vi "Main FPGA.vi"(7 "Motor Values":T3) -> ()   [LabVIEW 2013]
uses:
  <vilib>/rvi/Emulation/niFpgaSctlEmulationGetInTimedLoop.vi
  <vilib>/rvi/Emulation/niFpgaEmulationReportErrorSimple.vi
  <vilib>/rvi/Emulation/niFpgaGetClockAttributes.vi
  <vilib>/rvi/eio/common/nirviEmuTemplateMethod_errors.vi
  <vilib>/rvi/Emulation/niFpgaCriticalErrorInLSC.vi
  <vilib>/rvi/Emulation/niFpgaProcessEmulError.vi
  <vilib>/eio/EIONode/EIONode.xnode
panel:
  out "Data bit array":bool[](array[boolean])
  out "I2C FPGA Running":bool=TRUE
  in  "I2C Read":T1={"Data to send"=[0, 0, 0, 0, 0, 0, 0, 0], "Number of Bytes"=0, "Data to send 2"=[0, 0, 0, 0, 0, 0, 0, 0], "Number of Bytes 2"=0, "Data to send 3"=[0, 0, 0, 0, 0, 0, 0, 0], "Number of Bytes 3"=0, "Number of Bytes 4"=0, "I2C Start"=FALSE}
  in  "Position Reset 3":bool
  out "Position (Counts) 3":i16
  in  "Position Reset 2":bool
  out "Position (Counts) 2":i16
  out "Position (Counts)":i16
  in  "Position Reset":bool
  in  "Enable 4":bool
  in  "Encoder Intputs Motor 3":T2={"Tach 2"="ConnectorA/DIO9", "Tach 1"="ConnectorA/DIO8"}
  in  "Motor Values 3":T3
  in  "Motor Values 2":T3
  in  "Encoder Intputs Motor 2":T2={"Tach 2"="ConnectorB/DIO7", "Tach 1"="ConnectorB/DIO6"}
  in  "Encoder Intputs Motor 1":T2={"Tach 2"="ConnectorB/DIO9", "Tach 1"="ConnectorB/DIO8"}
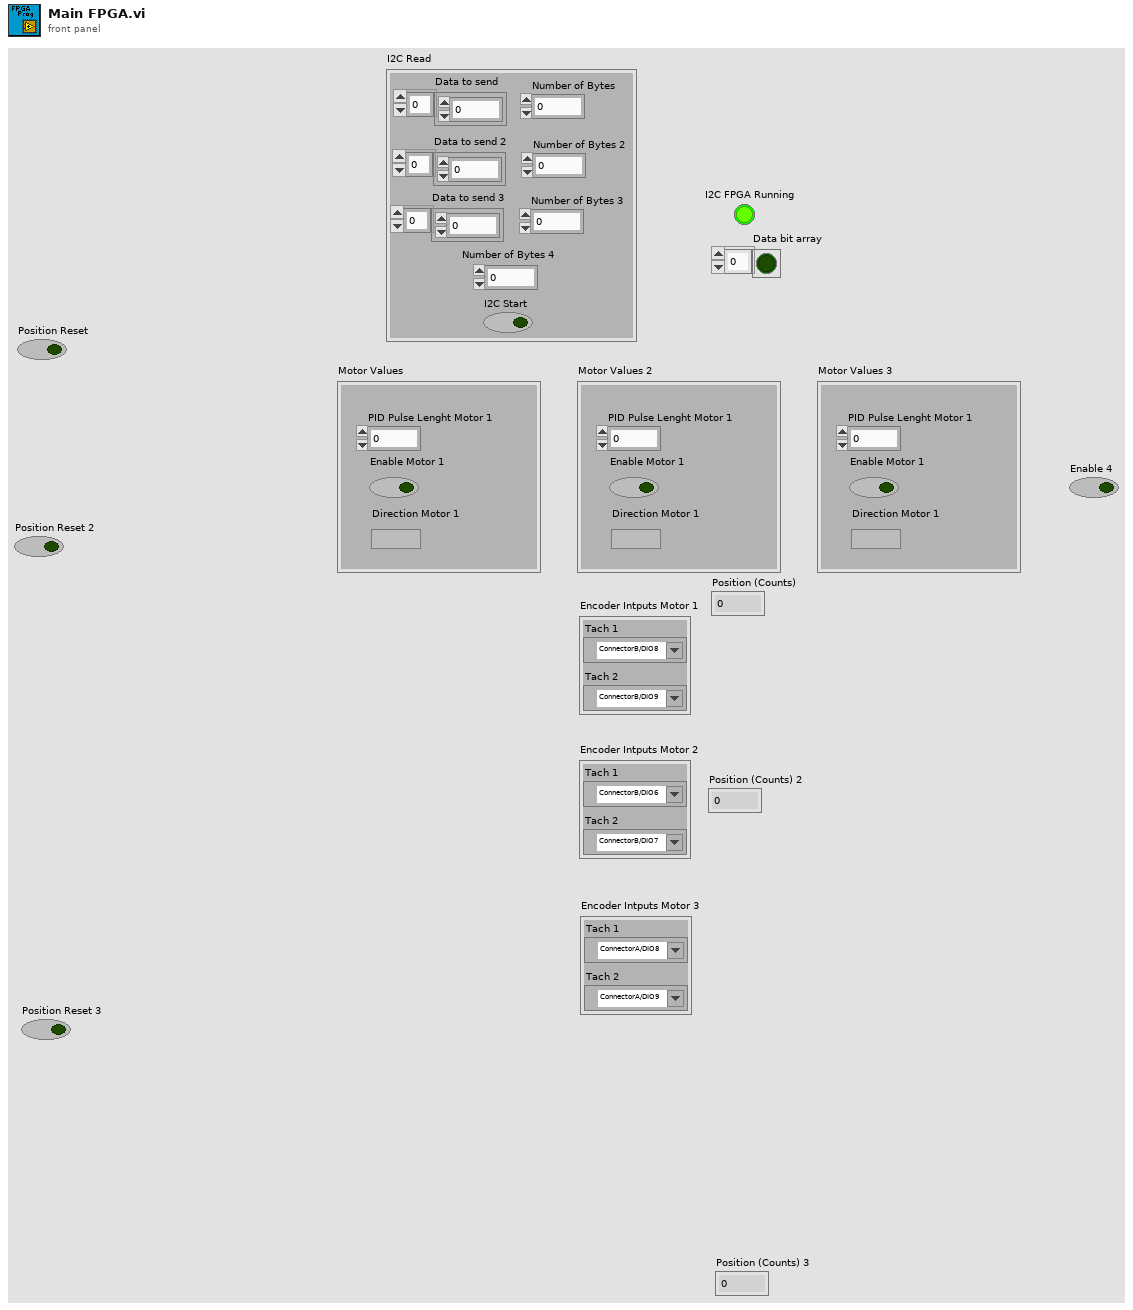
[diagram p1: front panel]
types:
  T1 = cluster{"Data to send":u8[], "Number of Bytes":i16, "Data to send 2":u8[], "Number of Bytes 2":i16, "Data to send 3":u8[], "Number of Bytes 3":i16, "Number of Bytes 4":i16, "I2C Start":bool}
  T2 = cluster{"Tach 2":refnum<k21>, "Tach 1":refnum<k21>}
  T3 = cluster{"PID Pulse Lenght Motor 1":i16, "Enable Motor 1":bool, "Direction Motor 1":bool}
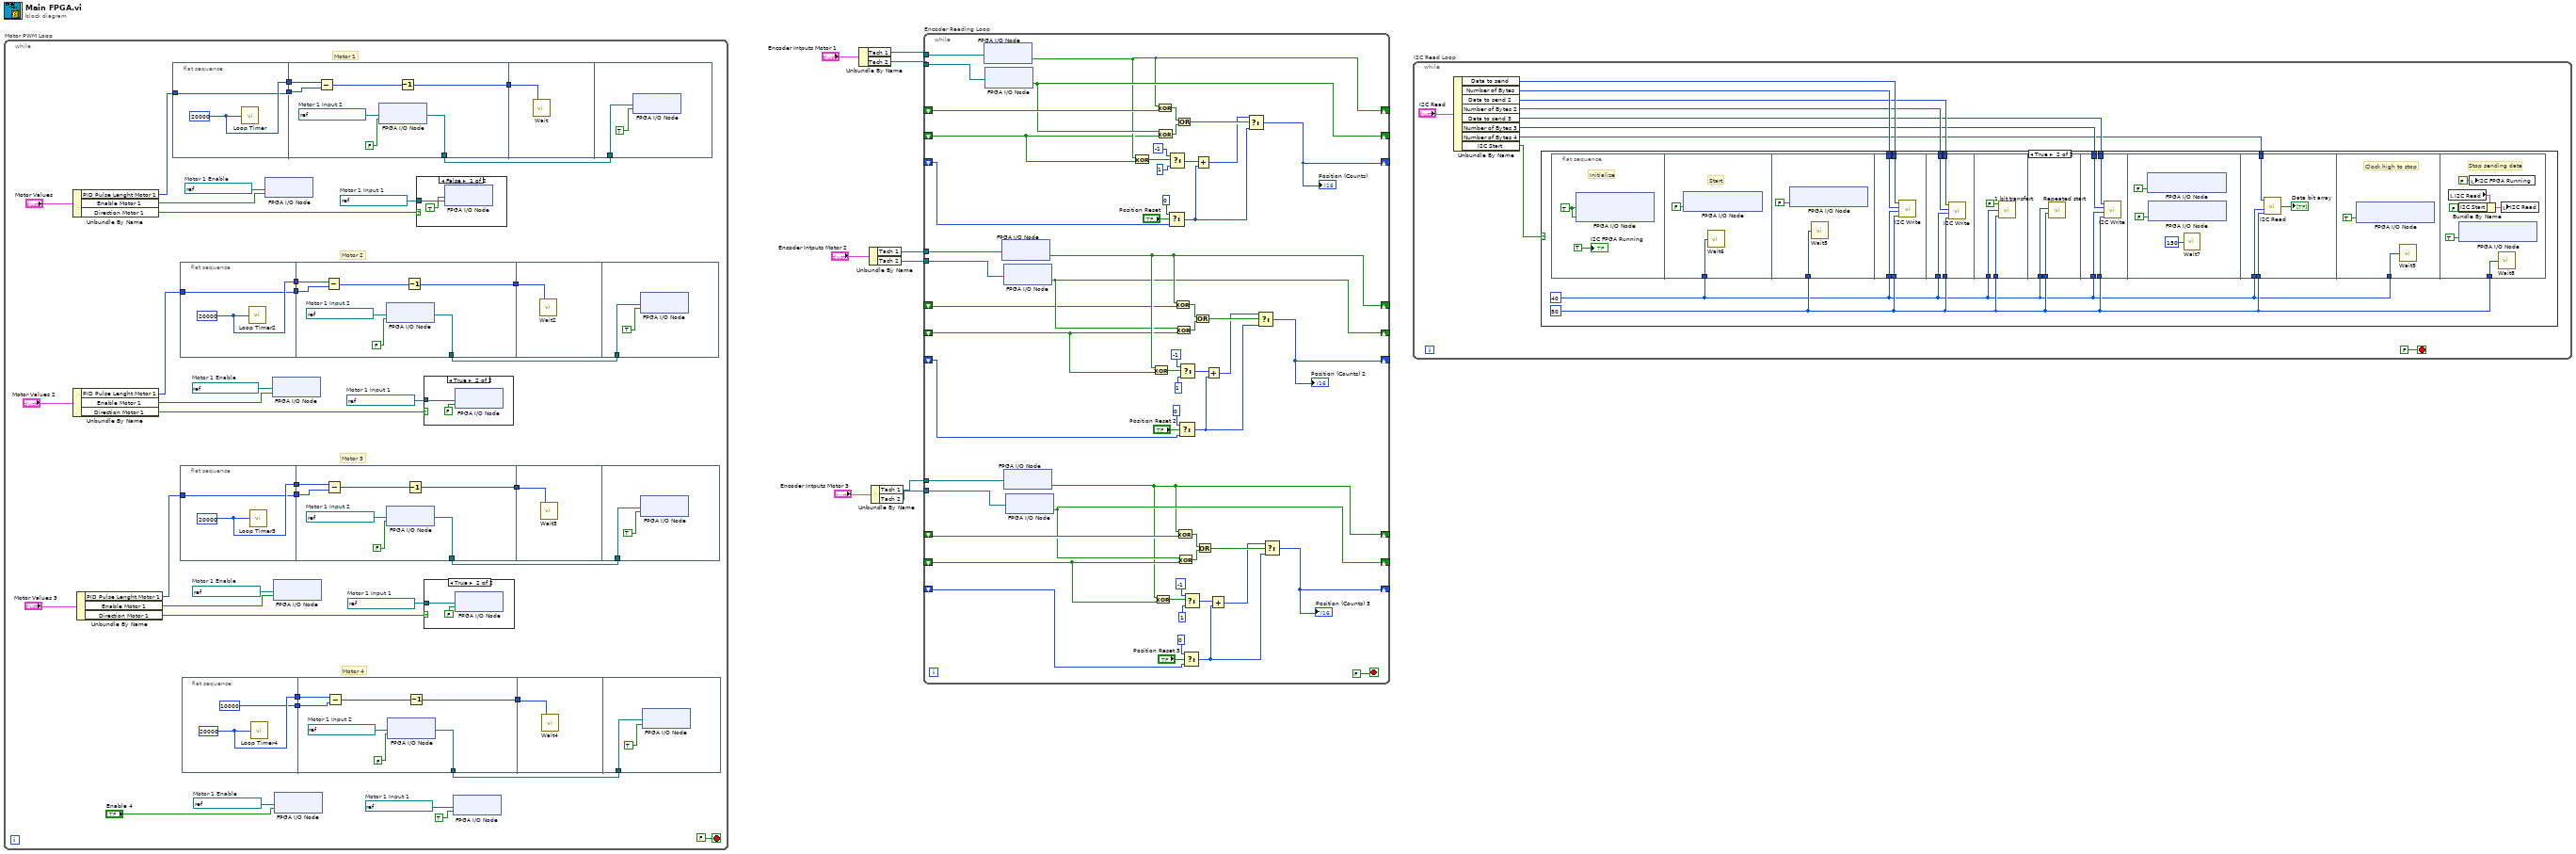
[diagram p0: block diagram]
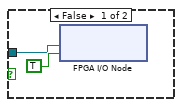
[diagram p3: hidden frame]
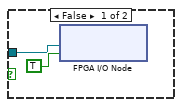
[diagram p4: hidden frame]
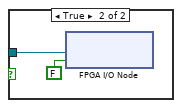
[diagram p5: hidden frame]
diagram:
  n1 = while "Motor PWM Loop" {
    stop <- FALSE stop-if-true
    w15 = refnum<k21> "ConnectorA/DIO1"  # Motor 1 Input 1
    w14 = refnum<k21> "ConnectorA/DIO0"  # Motor 1 Enable
    w22 = refnum<k21> "ConnectorA/DIO1"  # Motor 1 Input 1
    w23 = refnum<k21> "ConnectorA/DIO0"  # Motor 1 Enable
    w32 = refnum<k21> "ConnectorB/DIO4"  # Motor 1 Input 1
    w33 = refnum<k21> "ConnectorB/DIO3"  # Motor 1 Enable
    w42 = refnum<k21> "ConnectorB/DIO1"  # Motor 1 Input 1
    w43 = refnum<k21> "ConnectorB/DIO0"  # Motor 1 Enable
    # "Motor 4"
    # "Motor 3"
    # "Motor 2"
    # "Motor 1"
    n2 = Unbundle By Name("Motor Values") -> ("PID Pulse Lenght Motor 1"=w39:i16, "Enable Motor 1"=w41:bool, "Direction Motor 1"=w40:bool)
    n3 = Unbundle By Name("Motor Values 2") -> ("PID Pulse Lenght Motor 1"=w29:i16, "Enable Motor 1"=w31:bool, "Direction Motor 1"=w30:bool)
    n4 = Unbundle By Name("Motor Values 3") -> ("PID Pulse Lenght Motor 1"=w19:i16, "Enable Motor 1"=w21:bool, "Direction Motor 1"=w20:bool)
    n5 = flat-sequence {
      tunnel: [w98] -> w47
      tunnel: [w97] -> w46
      tunnel: w39 -> [w97]
      tunnel: [w105] -> w45
      tunnel: w47 -> [w104]
      tunnel: w46 -> [w103]
      tunnel: [w101] -> w44
      tunnel: w45 -> [w106]
      tunnel: w44 -> [w107]
      frame #0 {
        w98 = i16 20000
        n6 = call "Loop Timer"("Count(Ticks)"=w98) -> ()  [unwired: 1 out]
      }
      frame #1 {
        w99 = refnum<k21> "ConnectorB/DIO2"  # Motor 1 Input 2
        n7 = Subtract(x=w104, y=w103) -> (x-y=w102:i16)
        n8 = xnode "FPGA I/O Node"("I/O Item"=FALSE ("ConnectorC/DIO7"), "FPGA I/O In"=w99) -> ("FPGA I/O Out"=w101:refnum<k21>)
        n9 = Decrement(x=w102) -> (x-1=w105:i16)
      }
      frame #2 {
        n10 = call "Wait"("Count(Ticks)"=w106) -> ()  [unwired: 1 out]
      }
      frame #3 {
        n11 = xnode "FPGA I/O Node"("I/O Item"=TRUE ("ConnectorC/DIO7"), "FPGA I/O In"=w107) -> ()  [unwired: 1 out]
      }
    }
    n12 = flat-sequence {
      tunnel: [w82] -> w37
      tunnel: [w81] -> w36
      tunnel: w29 -> [w81]
      tunnel: [w89] -> w35
      tunnel: w37 -> [w88]
      tunnel: w36 -> [w87]
      tunnel: [w85] -> w34
      tunnel: w35 -> [w90]
      tunnel: w34 -> [w91]
      frame #0 {
        w82 = i16 20000
        n13 = call "Loop Timer2"("Count(Ticks)"=w82) -> ()  [unwired: 1 out]
      }
      frame #1 {
        w83 = refnum<k21> "ConnectorB/DIO5"  # Motor 1 Input 2
        n14 = Subtract(x=w88, y=w87) -> (x-y=w86:i16)
        n15 = xnode "FPGA I/O Node"("I/O Item"=FALSE ("ConnectorC/DIO7"), "FPGA I/O In"=w83) -> ("FPGA I/O Out"=w85:refnum<k21>)
        n16 = Decrement(x=w86) -> (x-1=w89:i16)
      }
      frame #2 {
        n17 = call "Wait2"("Count(Ticks)"=w90) -> ()  [unwired: 1 out]
      }
      frame #3 {
        n18 = xnode "FPGA I/O Node"("I/O Item"=TRUE ("ConnectorC/DIO7"), "FPGA I/O In"=w91) -> ()  [unwired: 1 out]
      }
    }
    n19 = flat-sequence {
      tunnel: [w66] -> w27
      tunnel: [w65] -> w26
      tunnel: w19 -> [w65]
      tunnel: [w73] -> w25
      tunnel: w27 -> [w72]
      tunnel: w26 -> [w71]
      tunnel: [w69] -> w24
      tunnel: w25 -> [w74]
      tunnel: w24 -> [w75]
      frame #0 {
        w66 = i16 20000
        n20 = call "Loop Timer3"("Count(Ticks)"=w66) -> ()  [unwired: 1 out]
      }
      frame #1 {
        w67 = refnum<k21> "ConnectorA/DIO2"  # Motor 1 Input 2
        n21 = Subtract(x=w72, y=w71) -> (x-y=w70:i16)
        n22 = xnode "FPGA I/O Node"("I/O Item"=FALSE ("ConnectorC/DIO7"), "FPGA I/O In"=w67) -> ("FPGA I/O Out"=w69:refnum<k21>)
        n23 = Decrement(x=w70) -> (x-1=w73:i16)
      }
      frame #2 {
        n24 = call "Wait3"("Count(Ticks)"=w74) -> ()  [unwired: 1 out]
      }
      frame #3 {
        n25 = xnode "FPGA I/O Node"("I/O Item"=TRUE ("ConnectorC/DIO7"), "FPGA I/O In"=w75) -> ()  [unwired: 1 out]
      }
    }
    n26 = flat-sequence {
      tunnel: [w50] -> w17
      tunnel: [i16 10000] -> w11
      tunnel: [w57] -> w16
      tunnel: w17 -> [w56]
      tunnel: [w54] -> w13
      tunnel: w11 -> [w51]
      tunnel: w16 -> [w58]
      tunnel: w13 -> [w59]
      frame #0 {
        w50 = i16 20000
        n27 = call "Loop Timer4"("Count(Ticks)"=w50) -> ()  [unwired: 1 out]
      }
      frame #1 {
        w52 = refnum<k21> "ConnectorA/DIO2"  # Motor 1 Input 2
        n28 = Subtract(x=w56, y=w51) -> (x-y=w55:i16)
        n29 = xnode "FPGA I/O Node"("I/O Item"=FALSE ("ConnectorC/DIO7"), "FPGA I/O In"=w52) -> ("FPGA I/O Out"=w54:refnum<k21>)
        n30 = Decrement(x=w55) -> (x-1=w57:i16)
      }
      frame #2 {
        n31 = call "Wait4"("Count(Ticks)"=w58) -> ()  [unwired: 1 out]
      }
      frame #3 {
        n32 = xnode "FPGA I/O Node"("I/O Item"=TRUE ("ConnectorC/DIO7"), "FPGA I/O In"=w59) -> ()  [unwired: 1 out]
      }
    }
    n33 = xnode "FPGA I/O Node"("I/O Item"=w41, "FPGA I/O In"=w43) -> ()  [unwired: 1 out]
    n34 = xnode "FPGA I/O Node"("I/O Item"=w31, "FPGA I/O In"=w33) -> ()  [unwired: 1 out]
    n35 = xnode "FPGA I/O Node"("I/O Item"=w21, "FPGA I/O In"=w23) -> ()  [unwired: 1 out]
    n36 = xnode "FPGA I/O Node"("I/O Item"="Enable 4", "FPGA I/O In"=w14) -> ()  [unwired: 1 out]
    n37 = case shown="False" w40 {
      tunnel: w42 -> [w93 w95]
      frame False {
        n38 = xnode "FPGA I/O Node"("I/O Item"=TRUE ("ConnectorC/DIO7"), "FPGA I/O In"=w93) -> ()  [unwired: 1 out]
      }
      frame True {
        n39 = xnode "FPGA I/O Node"("I/O Item"=FALSE ("ConnectorC/DIO7"), "FPGA I/O In"=w95) -> ()  [unwired: 1 out]
      }
    }
    n40 = case shown="True" w30 {
      tunnel: w32 -> [w77 w79]
      frame False {
        n41 = xnode "FPGA I/O Node"("I/O Item"=TRUE ("ConnectorC/DIO7"), "FPGA I/O In"=w77) -> ()  [unwired: 1 out]
      }
      frame True {
        n42 = xnode "FPGA I/O Node"("I/O Item"=FALSE ("ConnectorC/DIO7"), "FPGA I/O In"=w79) -> ()  [unwired: 1 out]
      }
    }
    n43 = case shown="True" w20 {
      tunnel: w22 -> [w61 w63]
      frame False {
        n44 = xnode "FPGA I/O Node"("I/O Item"=TRUE ("ConnectorC/DIO7"), "FPGA I/O In"=w61) -> ()  [unwired: 1 out]
      }
      frame True {
        n45 = xnode "FPGA I/O Node"("I/O Item"=FALSE ("ConnectorC/DIO7"), "FPGA I/O In"=w63) -> ()  [unwired: 1 out]
      }
    }
    n46 = xnode "FPGA I/O Node"("I/O Item"=TRUE ("ConnectorC/DIO7"), "FPGA I/O In"=w15) -> ()  [unwired: 1 out]
  }
  n47 = Unbundle By Name("Encoder Intputs Motor 1") -> ("Tach 1"=w8:refnum<k21>, "Tach 2"=w7:refnum<k21>)
  n48 = Unbundle By Name("Encoder Intputs Motor 2") -> ("Tach 1"=w5:refnum<k21>, "Tach 2"=w4:refnum<k21>)
  n49 = Unbundle By Name("Encoder Intputs Motor 3") -> ("Tach 1"=w2:refnum<k21>, "Tach 2"=w3:refnum<k21>)
  n50 = while "Encoder Reading Loop" {
    tunnel: w8 -> [w166]
    tunnel: w7 -> [w165]
    shift-right: [w160] -> _
    shift-left: _ -> [w162]
    shift-right: [w161] -> _
    shift-left: _ -> [w159]
    tunnel: w5 -> [w155]
    tunnel: w4 -> [w154]
    shift-right: [w153] -> _
    shift-left: _ -> [w151]
    shift-right: [w152] -> _
    shift-left: _ -> [w150]
    tunnel: w2 -> [w144]
    tunnel: w3 -> [w145]
    shift-right: [w146] -> _
    shift-left: _ -> [w148]
    shift-right: [w147] -> _
    shift-left: _ -> [w149]
    shift-right: [w136] -> _
    shift-left: _ -> [w132]
    shift-right: [w124] -> _
    shift-left: _ -> [w120]
    shift-right: [w110] -> _
    shift-left: _ -> [w109]
    stop <- FALSE stop-if-true
    n51 = xnode "FPGA I/O Node"("FPGA I/O In"=w166) -> ("I/O Item"=w160:bool)  [unwired: 1 out]
    n52 = xnode "FPGA I/O Node"("FPGA I/O In"=w165) -> ("I/O Item"=w161:bool)  [unwired: 1 out]
    n53 = xnode "FPGA I/O Node"("FPGA I/O In"=w155) -> ("I/O Item"=w153:bool)  [unwired: 1 out]
    n54 = xnode "FPGA I/O Node"("FPGA I/O In"=w154) -> ("I/O Item"=w152:bool)  [unwired: 1 out]
    n55 = xnode "FPGA I/O Node"("FPGA I/O In"=w144) -> ("I/O Item"=w146:bool)  [unwired: 1 out]
    n56 = xnode "FPGA I/O Node"("FPGA I/O In"=w145) -> ("I/O Item"=w147:bool)  [unwired: 1 out]
    n57 = Exclusive Or(1:w159, 2:w160) -> (0:w140:bool)
    n58 = Exclusive Or(1:w150, 2:w153) -> (0:w126:bool)
    n59 = Exclusive Or(1:w149, 2:w146) -> (0:w114:bool)
    n60 = Exclusive Or(1:w162, 2:w160) -> (0:w163:bool)
    n61 = Exclusive Or(1:w159, 2:w161) -> (0:w164:bool)
    n62 = Select(t=i16 0, s="Position Reset", f=w132) -> (s? t:f=w135:i16)
    n63 = Select(t=i16 -1, s=w140, f=i16 1) -> (s? t:f=w139:i16)
    n64 = Exclusive Or(1:w151, 2:w153) -> (0:w157:bool)
    n65 = Exclusive Or(1:w150, 2:w152) -> (0:w156:bool)
    n66 = Or(x=w163, y=w164) -> (x .or. y?=w141:bool)
    n67 = Exclusive Or(1:w148, 2:w146) -> (0:w142:bool)
    n68 = Exclusive Or(1:w149, 2:w147) -> (0:w143:bool)
    n69 = Select(t=i16 0, s="Position Reset 2", f=w120) -> (s? t:f=w122:i16)
    n70 = Select(t=i16 -1, s=w126, f=i16 1) -> (s? t:f=w127:i16)
    n71 = Select(t=i16 0, s="Position Reset 3", f=w109) -> (s? t:f=w112:i16)
    n72 = Select(t=i16 -1, s=w114, f=i16 1) -> (s? t:f=w118:i16)
    n73 = Or(x=w157, y=w156) -> (x .or. y?=w125:bool)
    n74 = Add(x=w139, y=w135) -> (x+y=w138:i16)
    n75 = Or(x=w142, y=w143) -> (x .or. y?=w113:bool)
    n76 = Add(x=w127, y=w122) -> (x+y=w123:i16)
    n77 = Add(x=w118, y=w112) -> (x+y=w111:i16)
    n78 = Select(t=w138, s=w141, f=w135) -> (s? t:f=w136:i16)
    "Position (Counts)" <- w136
    n79 = Select(t=w123, s=w125, f=w122) -> (s? t:f=w124:i16)
    "Position (Counts) 2" <- w124
    n80 = Select(t=w111, s=w113, f=w112) -> (s? t:f=w110:i16)
    "Position (Counts) 3" <- w110
  }
  n81 = while "I2C Read Loop" {
    stop <- FALSE stop-if-true
    n82 = Unbundle By Name("I2C Read") -> ("Data to send"=w174:u8[], "Number of Bytes"=w173:i16, "Data to send 2"=w172:u8[], "Number of Bytes 2"=w171:i16, "Data to send 3"=w170:u8[], "Number of Bytes 3"=w169:i16, "Number of Bytes 4"=w168:i16, "I2C Start"=w167:bool)
    n83 = case shown="True" w167 {
      tunnel: w174 -> [_ w185]
      tunnel: w173 -> [_ w184]
      tunnel: w172 -> [_ w181]
      tunnel: w171 -> [_ w180]
      tunnel: w170 -> [_ w179]
      tunnel: w169 -> [_ w178]
      tunnel: w168 -> [_ w177]
      frame False {
      }
      frame True {
        w183 = u32 50 ("Min time SCl low (uSec)")
        w182 = u32 40 ("Min Time SCL high (uSec)")
        n84 = flat-sequence {
          tunnel: w182 -> [w188]
          tunnel: w183 -> [w190]
          tunnel: w183 -> [w195]
          tunnel: w182 -> [w194]
          tunnel: w185 -> [w193]
          tunnel: w184 -> [w192]
          tunnel: w183 -> [w199]
          tunnel: w182 -> [w198]
          tunnel: w181 -> [w197]
          tunnel: w180 -> [w196]
          tunnel: w183 -> [w201]
          tunnel: w182 -> [w200]
          tunnel: w183 -> [w204]
          tunnel: w182 -> [w203]
          tunnel: w183 -> [w208]
          tunnel: w182 -> [w207]
          tunnel: w179 -> [w206]
          tunnel: w178 -> [w205]
          tunnel: w183 -> [w215]
          tunnel: w182 -> [w214]
          tunnel: w177 -> [w213]
          tunnel: w182 -> [w216]
          tunnel: w183 -> [w222]
          frame #0 {
            w187 = TRUE ("ConnectorC/DIO1")
            # "Initialize"
            n85 = xnode "FPGA I/O Node"("ConnectorB/DIO13"=w187, "ConnectorB/DIO12"=w187) -> ()  [unwired: 2 in, 2 out]
            "I2C FPGA Running" <- TRUE ("FPGA Running")
          }
          frame #1 {
            # "Start"
            n86 = xnode "FPGA I/O Node"("ConnectorB/DIO13"=FALSE ("ConnectorC/DIO1")) -> ()  [unwired: 1 in, 1 out]
            n87 = call "Wait6"("Count(uSec)"=w188) -> ()  [unwired: 1 out]
          }
          frame #2 {
            n88 = xnode "FPGA I/O Node"("ConnectorB/DIO12"=FALSE ("ConnectorC/DIO0")) -> ()  [unwired: 1 in, 1 out]
            n89 = call "Wait5"("Count(uSec)"=w190) -> ()  [unwired: 1 out]
          }
          frame #3 {
            n90 = call "I2C Write.vi"("Min time SCL low (uSec)"=w195, "Min Time SCL high (uSec)"=w194, "Number of Bytes"=w192, "Data to send"=w193) -> ()  [unwired: 1 in]
          }
          frame #4 {
            n91 = call "I2C Write.vi"("Min time SCL low (uSec)"=w199, "Min Time SCL high (uSec)"=w198, "Number of Bytes"=w196, "Data to send"=w197) -> ()  [unwired: 1 in]
          }
          frame #5 {
            n92 = call "1 bit transfert.vi"("Min time SCL low (uSec)"=w201, "Min Time SCL high (uSec)"=w200, "Data bit"=FALSE) -> ()  [unwired: 1 in]
          }
          frame #6 {
            n93 = call "Repeated start.vi"("Min time SCL low (uSec)"=w204, "Min time SCL high (uSec)"=w203) -> ()  [unwired: 10 in]
          }
          frame #7 {
            n94 = call "I2C Write.vi"("Min time SCL low (uSec)"=w208, "Min Time SCL high (uSec)"=w207, "Number of Bytes"=w205, "Data to send"=w206) -> ()  [unwired: 1 in]
          }
          frame #8 {
            n95 = xnode "FPGA I/O Node"("ConnectorB/DIO12"=FALSE ("ConnectorC/DIO0")) -> ()  [unwired: 1 in, 1 out]
            n96 = xnode "FPGA I/O Node"("ConnectorB/DIO13"=FALSE ("ConnectorC/DIO0")) -> ()  [unwired: 1 in, 1 out]
            n97 = call "Wait7"("Count(uSec)"=u32 150) -> ()  [unwired: 1 out]
          }
          frame #9 {
            n98 = call "I2C Read.vi"("Min time SCl low (uSec)"=w215, "Min Time SCL high (uSec)"=w214, "Number of Bytes"=w213) -> ("Data bit array"=→"Data bit array":bool[])  [unwired: 1 in]
          }
          frame #10 {
            # "Clock high to stop"
            n99 = xnode "FPGA I/O Node"("ConnectorB/DIO12"=TRUE ("ConnectorC/DIO0")) -> ()  [unwired: 1 in, 1 out]
            n100 = call "Wait9"("Count(uSec)"=w216) -> ()  [unwired: 1 out]
          }
          frame #11 {
            # "Stop sending data"
            n101 = local read "I2C Read"() -> (w219:T1)
            n102 = xnode "FPGA I/O Node"("ConnectorB/DIO13"=TRUE ("ConnectorC/DIO0")) -> ()  [unwired: 1 in, 1 out]
            n103 = Bundle By Name(cluster=w219, "I2C Start"=FALSE) -> (w218:T1)
            n104 = local write "I2C FPGA Running"(FALSE) -> ()
            n105 = call "Wait8"("Count(uSec)"=w222) -> ()  [unwired: 1 out]
            n106 = local write "I2C Read"(w218) -> ()
          }
        }
      }
    }
  }
